vi "Check Status.vi"(8 "error in (no error)":errorcluster, 11 "Temperature Controller in":refnum<class "Temperature Controller.lvclass">) -> (0 "error out":errorcluster, 1 "Status":string, 2 "Ready?":bool, 3 "Temperature Controller out":refnum<class "Temperature Controller.lvclass">)   [LabVIEW 2023, in "Temperature Controller.lvclass"]
doc: "(Dynamic) Check if the instrument is powered on and update its member fields with the instrument's current status. Optionally return a text status message."
uses:
  Temperature Controller.lvclass
  Temperature Controller.lvclass/Temperature Controller.ctl
panel:
  out "Ready? 2":bool
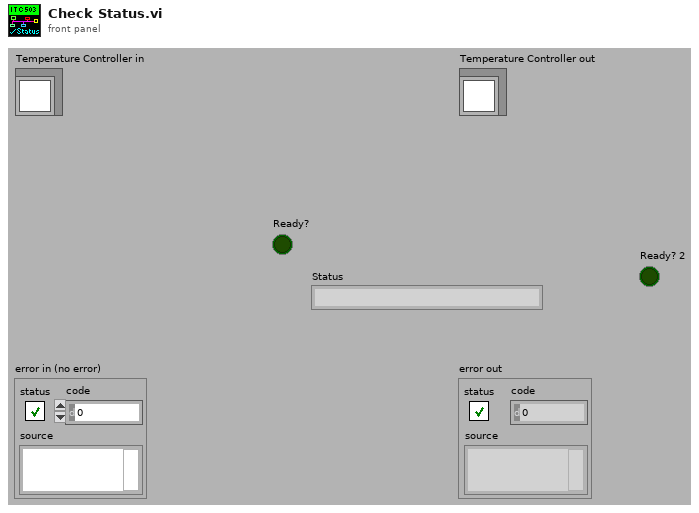
[diagram p1: front panel]
types:
  T1 = typedef "OxfordAddress.ctl" = cluster{"Com Port":i32, "ISOBUS Address":i32, "GPIB Address":i16, "Communication":enum16{"RS232", "ISOBUS", "GPIB", "Gateway"}}
  T2 = typedef "Temperature Controller.lvclass/HV Slide Indicator.ctl" = dbl
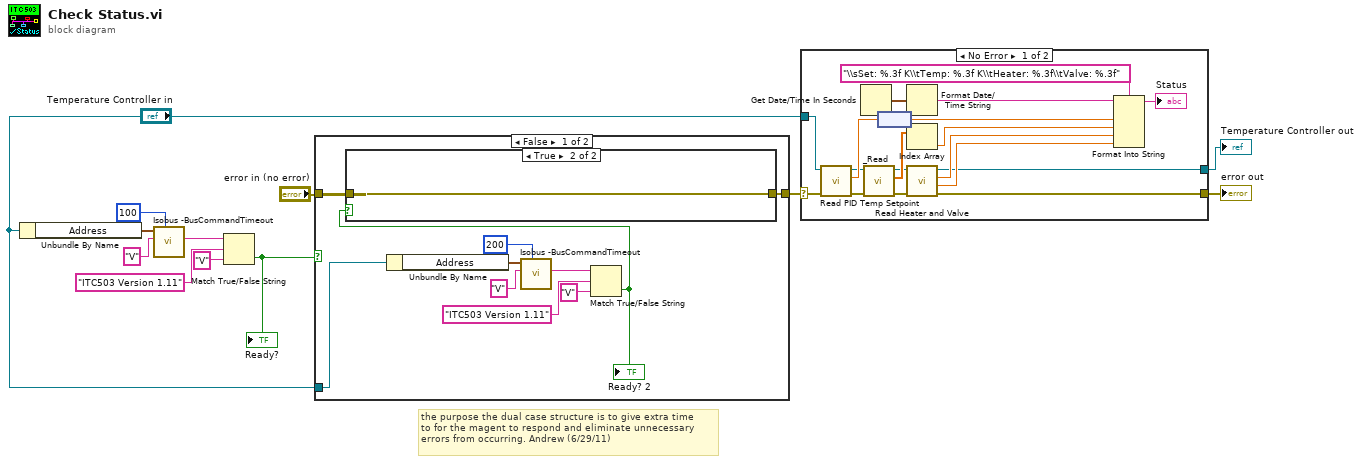
[diagram p0: block diagram]
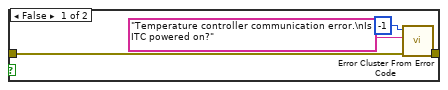
[diagram p2: hidden frame]
diagram:
  # "the purpose the dual case structure is to give extra time\nto for the magent to respond and eliminate unnecessary\nerrors from occurring. Andrew (6/29/11)"
  n1 = Unbundle By Name("Temperature Controller in") -> ("Address"=w4:T1)
  n2 = call "Isobus -BusCommandTimeout.vi"("Timeout (ms)"=100, "Command"="V", "Address"=w4) -> ("Reply"=w2:string)  [unwired: 5 out]
  n3 = Match True/False String(2:"V", 3:"ITC503 Version 1.11", 4:w2) -> (0:w6:bool)  [unwired: 1 out]
  "Ready?" <- w6
  n4 = case shown="False" w6 {
    tunnel: "error in (no error)" -> [w22 w28]
    tunnel: [w21 w28] -> w9
    tunnel: "Temperature Controller in" -> [w13 _]
    frame False {
      n5 = Unbundle By Name(w13) -> ("Address"=w18:T1)
      n6 = call "Isobus -BusCommandTimeout.vi"("Timeout (ms)"=200, "Command"="V", "Address"=w18) -> ("Reply"=w20:string)  [unwired: 5 out]
      n7 = Match True/False String(2:"V", 3:"ITC503 Version 1.11", 4:w20) -> (0:w14:bool)  [unwired: 1 out]
      "Ready? 2" <- w14
      n8 = case shown="True" w14 {
        tunnel: w22 -> [w24 w27]
        tunnel: [w23 w27] -> w21
        frame False {
          n9 = call <vilib>:"Error Cluster From Error Code.vi"("error in (no error)"=w24, "error message (\"\")"="Temperature controller communication error.\nIs ITC powered on?" ("error message (\"\")"), "error code (0)"=-1) -> ("error out"=w23:errorcluster)  [unwired: 6 in]
        }
        frame True {
        }
      }
    }
    frame True {
    }
  }
  n10 = case shown="No Error" w9 {
    selector: w9 -> [w37 w48]
    tunnel: [w32 w47] -> w12
    tunnel: "Temperature Controller in" -> [w36 w47]
    tunnel: [w33 w48] -> w11
    frame No Error {
      n11 = call-dynamic "Read PID Temp Setpoint.vi"("error in (no error)"=w37, "Temperature Controller in"=w36) -> ("error out"=w34:errorcluster, "PID Temp Setpoint"=w38:dbl[unit], "Temperature Controller out"=w35:refnum<class "Temperature Controller.lvclass">)  [unwired: 7 in]
      n12 = Get Date/Time In Seconds() -> (seconds since 1Jan1904=w31:timestamp)
      n13 = call-dynamic "_Read.vi"("error in (no error)"=w34, "Temperature Controller.lvclass"=w35) -> ("error out"=w40:errorcluster, "Data Points"=w44:dbl[], "Temperature Controller out"=w43:refnum<class "Temperature Controller.lvclass">)  [unwired: 7 in]
      n14 = node(w38) -> (w29:dbl)
      n15 = Format Date/Time String(seconds (now)=w31) -> (date/time string=w30:string)  [unwired: 2 in]
      n16 = Index Array(array=w44) -> (element=w39:dbl)  [unwired: 1 in]
      n17 = call-dynamic "Read Heater and Valve.vi"("error in (no error)"=w40, "Temperature Controller in"=w43) -> ("error out"=w33:errorcluster, "valve%"=w41:T2, "heater%"=w42:T2, "Temperature Controller out"=w32:refnum<class "Temperature Controller.lvclass">)  [unwired: 6 in]
      n18 = Format Into String(format string="\\sSet: %.3f K\\tTemp: %.3f K\\tHeater: %.3f\\tValve: %.3f", initial string=w30, w29, w39, w42, w41) -> (resulting string=→"Status":string)  [unwired: 1 in, 1 out]
    }
    frame Error {
    }
  }
  "error out" <- w11
  "Temperature Controller out" <- w12
